vi "Find next DIT & return elements.vi"(0 "Text & DIT(s)":string="Now is the time for all good men to come to the aid of their country.\n<DIT><Coded Hash=xxxxx><Public=xxxxx><n=xxxxx></DIT>", 11 "error in (no error)":errorcluster) -> (2 "Special DIT?":bool, 3 "DIT found?":bool, 4 "Text before DIT":string, 6 "Decoded Hash value (HEX)":string="ÿÿÿÿ", 8 "Text after DIT":string, 10 "Public Key (Hex)":string, 14 "n (Hex)":string="ÿÿÿÿ", 15 "error out":errorcluster)   [LabVIEW 2009]
doc: "Searches from the beginning of the string for a complete DIT tag. If found, it returns the tag elements, the string before and the string after the tag.\n\nFormat of tag\n<DIT><Coded Hash=xxxxx><Public=xxxxx><n=xxxxx></DIT>\n\nThe xxxx values are acsii coded strings and must be converted to hex strings before processing."
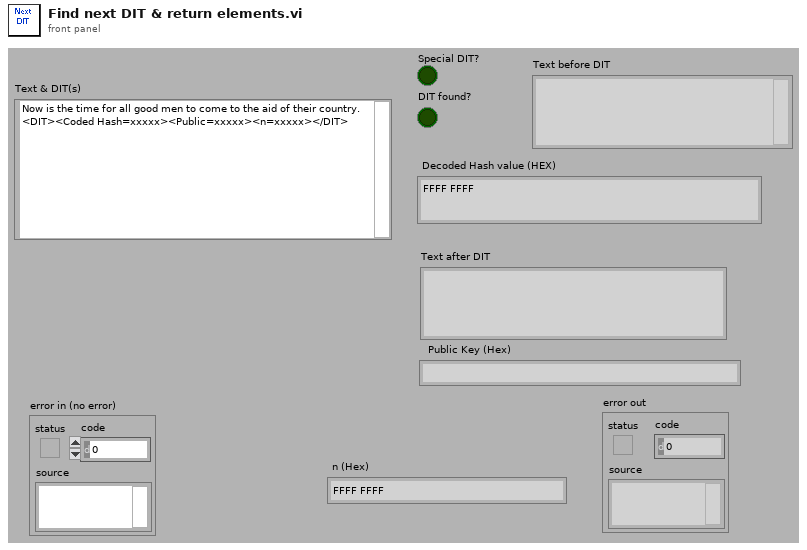
[diagram p1: front panel]
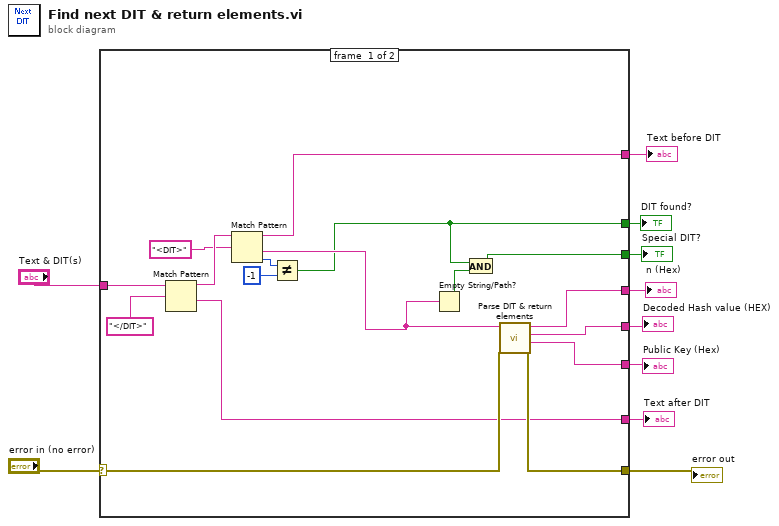
[diagram p0: block diagram]
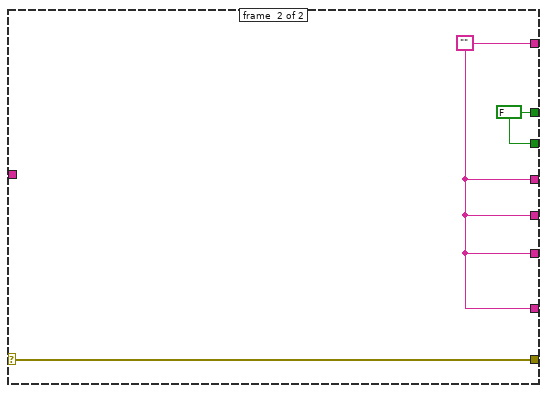
[diagram p2: hidden frame]
diagram:
  n1 = case shown="No Error" "error in (no error)" {
    selector: "error in (no error)" -> [w24 w30]
    tunnel: [w23 w30] -> w9
    tunnel: [w27 w29] -> w8
    tunnel: [w26 w29] -> w7
    tunnel: [w25 w29] -> w6
    tunnel: "Text & DIT(s)" -> [w22 _]
    tunnel: [w19 w29] -> w4
    tunnel: [w17 w29] -> w3
    tunnel: [w13 w28] -> w2
    tunnel: [w11 w28] -> w1
    frame #0 {
      n2 = Match Pattern(string=w22, regular expression="</DIT>" ("String")) -> (before substring=w20:string, after substring=w19:string)  [unwired: 3 out]
      n3 = Match Pattern(string=w20, regular expression="<DIT>" ("String")) -> (before substring=w17:string, after substring=w14:string, offset past match=w16:i32)  [unwired: 2 out]
      n4 = Not Equal?(x=w16, y=-1) -> (x != y?=w13:bool)
      n5 = Empty String/Path?(string/path=w14) -> (empty?=w12:bool)
      n6 = And(x=w13, y=w12) -> (x .and. y?=w11:bool)
      n7 = call "Parse DIT & return elements.vi"("error in (no error)"=w24, "DIT string"=w14) -> ("error out"=w23:errorcluster, "Public Key (Hex)"=w25:string, "Decoded Hash value (Hex)"=w26:string, "n (Hex)"=w27:string)  [unwired: 6 out]
    }
    frame #1 {
      w28 = FALSE
      w29 = ""
    }
  }
  "n (Hex)" <- w8
  "error out" <- w9
  "Public Key (Hex)" <- w6
  "Text before DIT" <- w3
  "Decoded Hash value (HEX)" <- w7
  "Text after DIT" <- w4
  "DIT found?" <- w2
  "Special DIT?" <- w1
